vi "Update-mapping-vars.vi"(8 "error in":errorcluster, 11 "Data ref. in":refnum<data-value>) -> (0 "error IO":errorcluster, 3 "Data ref.":refnum<data-value>)   [LabVIEW 2013, in "CameraVision.lvlib" / "CV-Main.lvclass"]
doc: "If the 'Mapping' option is enabled, this function loads the scan pattern information file into memory and translates the laser commands into time-x-y and laser on/off data. This data is later used to correlate with the time-characteristic data to form an x-y-characteristic 3D color graph.\n\nThis function is only a wrapper for the actual scan pattern parser, which allows to quickly update the (cross-application) parser to a new version without breaking functionality."
uses:
  CV-Main.lvclass
  CV-Main.lvclass/CV-Main.ctl
  Mapping/CV-Mapping.lvclass/CV-Mapping.ctl
  UI/Module-states.ctl
  Mapping/Write Time.vi
  Mapping/Write Xcoors.vi
  Mapping/Write Ycoors.vi
  Mapping/Write Scan start.vi
  Mapping/Write Mapping offset.vi
  Mapping/Write Mapping status.vi
  Mapping/Read Enable mapping.vi
  Mapping/Read Scan pattern file.vi
  Mapping/Read Default mark speed.vi
  Mapping/Read Jump speed.vi
  Read Mapping params.vi
  Mapping/CV-Mapping.lvclass
  UI/CV-UI.lvclass
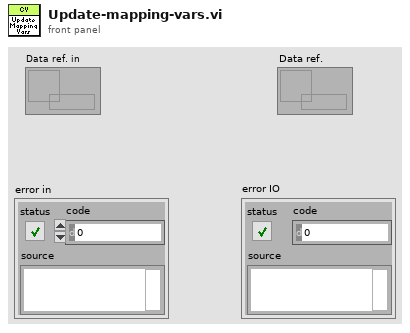
[diagram p1: front panel]
types:
  T1 = typedef "CameraVision.lvlib/CV-UI.lvclass/Module-states.ctl" = enum16{"Inactive", "Active", "Data-loss", "Error", "Simulation", "Synchronizing", "Initialized", "Released"}
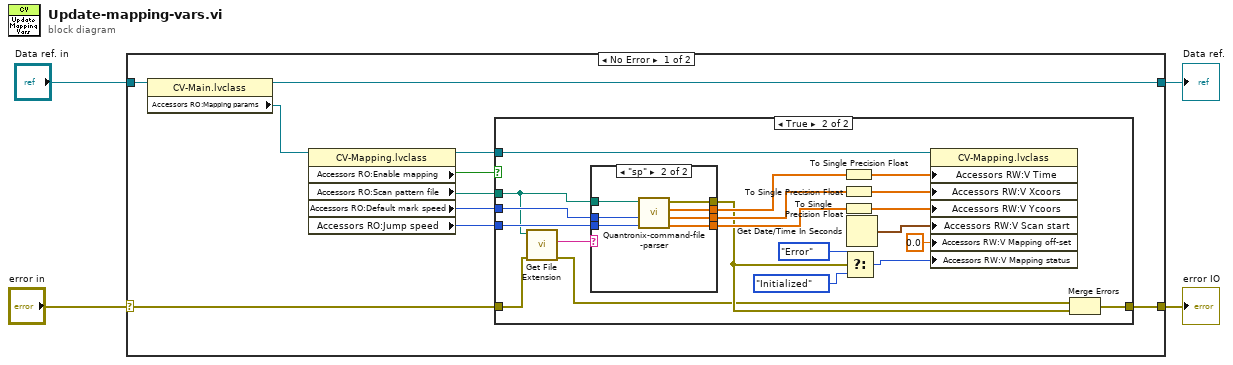
[diagram p0: block diagram]
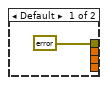
[diagram p3: hidden frame]
diagram:
  n1 = case shown="No Error" "error in" {
    selector: "error in" -> [w7 w45]
    tunnel: [w14 w45] -> w3
    tunnel: "Data ref. in" -> [w8 w44]
    tunnel: [w6 w44] -> w1
    frame No Error {
      n2 = property class="CV-Main.lvclass"(reference=w8) -> (reference out=w6:refnum<data-value>, "Accessors RO:Mapping params"=w5:refnum<data-value>)  [unwired: 1 in, 1 out]
      n3 = property class="CV-Mapping.lvclass"(reference=w5) -> (reference out=w9:refnum<data-value>, "Accessors RO:Enable mapping"=w13:bool, "Accessors RO:Scan pattern file"=w12:path, "Accessors RO:Default mark speed"=w11:i32, "Accessors RO:Jump speed"=w10:i32)  [unwired: 1 in, 1 out]
      n4 = case shown="True" w13 {
        tunnel: [w15 w32] -> w14
        tunnel: w12 -> [_ w29]
        tunnel: w11 -> [_ w31]
        tunnel: w10 -> [_ w30]
        tunnel: w7 -> [w15 w28]
        tunnel: w9 -> [_ w22]
        frame False {
        }
        frame True {
          n5 = call <vilib>:"Get File Extension.vi"("error in (no error)"=w28, "file"=w29) -> ("error out"=w23:errorcluster, "lowercase file extension"=w27:string)  [unwired: 6 in, 2 out]
          n6 = case shown="\"sp\"" w27 {
            tunnel: [_ w43] -> w35
            tunnel: [_ w42] -> w34
            tunnel: [_ w41] -> w33
            tunnel: w31 -> [_ w40]
            tunnel: w30 -> [_ w39]
            tunnel: [errorcluster {"status"=TRUE, "code"=0, "source"="Mapping: unrecongized file extension."} ("error out") w38] -> w24
            tunnel: w29 -> [_ w37]
            frame Default {
            }
            frame "sp" {
              n7 = call "Quantronix-command-file-parser.vi"("Move speed [mm/s]"=w39, "Scan speed [mm/s]"=w40, "Scan pattern file path"=w37) -> ("Ycoors"=w41:dbl[], "Xcoors"=w42:dbl[], "Time"=w43:dbl[], "error out"=w38:errorcluster)  [unwired: 2 in, 3 out]
            }
          }
          n8 = To Single Precision Float(number=w35) -> (single precision float=w21:sgl[])
          n9 = To Single Precision Float(number=w34) -> (single precision float=w20:sgl[])
          n10 = To Single Precision Float(number=w33) -> (single precision float=w19:sgl[])
          n11 = Select(t=Module-states."Error" ("Mapping status"), s=w24, f=Module-states."Initialized" ("Mapping status")) -> (s? t:f=w17:T1)
          n12 = Get Date/Time In Seconds() -> (seconds since 1Jan1904=w16:timestamp)
          n13 = property class="CV-Mapping.lvclass"(reference=w22, "Accessors RW:V Time"=w21, "Accessors RW:V Xcoors"=w20, "Accessors RW:V Ycoors"=w19, "Accessors RW:V Scan start"=w16, "Accessors RW:V Mapping off-set"=0.0 ("V Mapping off-set"), "Accessors RW:V Mapping status"=w17) -> ()  [unwired: 1 in, 2 out]
          n14 = Merge Errors(w23, w24) -> (w32:errorcluster)
        }
      }
    }
    frame Error {
    }
  }
  "error IO" <- w3
  "Data ref." <- w1
